vi "Com_Panel_Panel Close.vi"(8 "error in":errorcluster, 11 "VI Refnum In":refnum<vi>) -> (0 "error out":errorcluster, 3 "VI Refnum Out":refnum<vi>)   [LabVIEW 2016]
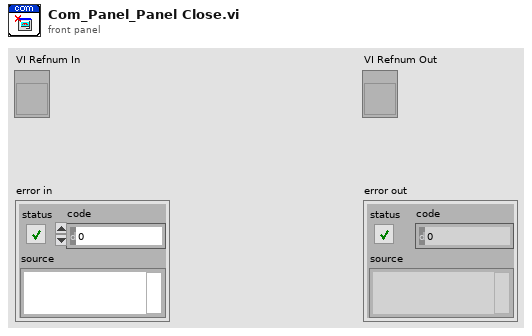
[diagram p1: front panel]
types:
  T1 = enum32{"Invalid", "Standard", "Closed", "Hidden", "Minimized", "Maximized"}
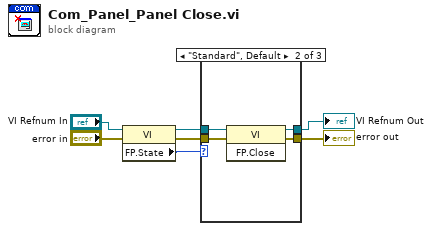
[diagram p0: block diagram]
diagram:
  n1 = property class="VI"(reference="VI Refnum In", error in="error in") -> (reference out=w5:refnum<vi>, error out=w6:errorcluster, "FP.State"=w7:T1)
  n2 = case shown="\"Standard\", Default" w7 {
    tunnel: [w9 w13 w15] -> w4
    tunnel: [w8 w12 w14] -> w3
    tunnel: w6 -> [w9 w11 w15]
    tunnel: w5 -> [w8 w10 w14]
    frame "Invalid" {
    }
    frame "Standard", Default {
      n3 = invoke class="VI" method="FP.Close"(reference=w10, error in=w11) -> (reference out=w12:refnum<vi>, error out=w13:errorcluster)  [unwired: 1 in, 1 out]
    }
    frame "Closed" {
    }
  }
  "VI Refnum Out" <- w3
  "error out" <- w4
